vi "AlliGator Highlight Phasor ROI in Original Image v3.vi"(0 "AlliGator IV DVR in":refnum<data-value>, 1 "Image Color Scale Information":T2, 2 "Temp Overlay?":bool, 5 "Source Image Display":T1, 7 "Phasor Plot Image":T1, 9 "Phasor Plot ROI":T3, 11 "Error In":errorcluster, 12 "Overlay Color":u32(colorbox)) -> (4 "AlliGator IV DVR out":refnum<data-value>, 6 "Source Image Display out":T1, 8 "Phasor Plot Image Out":T1, 14 "CPU (s)":dbl, 15 "Error Out":errorcluster)   [LabVIEW 2021, in "AlliGator Source Image.lvlib"]
doc: "Compute and overlays the selected Phasor Plot ROI's pixels in the Source Image."
uses:
  AlliGator Source Image.lvlib
  AlliGator Internal Variables v2.ctl
  <vilib>/vision/Image Controls.llb/IMAQ Image.ctl
  AlliGator Gate Image Set.ctl
  AlliGator FLI Dataset Type.ctl
  AlliGator Data Series Type.ctl
  AlliGator Dataset Channel.ctl
  AlliGator Gate Arithmetic.ctl
  AlliGator Displayed Image.ctl
  Image/Named ROI Description.ctl
  AlliGator Decay Metadata v3.ctl
  AlliGator Decay Background Subtraction Info.ctl
  AlliGator Baseline Subtraction Method.ctl
  Graphs/XY Graph/XY Graph Plot Shift Parameters.ctl
  Graphs/XY Graph/XY Graph Plot Shift Method.ctl
  AlliGator Decay Extrapolation Parameters.ctl
  Phasor/Calibration Phasor (m, phi).ctl
  Phasor/Phasor Reference Series.ctl
  Phasor/Phasor Calibration Map v2.ctl
  Phasor/Phasor (g, s).ctl
  AlliGator Raw Phasor Plot Data v4.ctl
  Phasor/Phasor Standard Deviation Options.ctl
  AlliGator Phasor Multi-Harmonic Data.ctl
  Phasor/Phasor Harmonic Data.ctl
  AlliGator Decay Fit Options & Parameters v2.ctl
  Fits/IRF(X)PSED/Decay Fit Options v2.ctl
  Fits/Decay Convolution/Decay Model.ctl
  Fits/Residual Type.ctl
  Fits/IRF(X)PSED/Fit Weights Type.ctl
  Fits/Non-linear Fitting Method v2.ctl
  Fits/Fit Calculation Method.ctl
  Fits/Non-linear Fitting Algorithm.ctl
  AlliGator Decay Fit Parameter Constraints 2.ctl
  Fits/IRF(X)PSED/Decay Fit Parameters In List.ctl
  Fits/IRF(X)PSED/MLE Baseline Offset Type.ctl
  AlliGator Decay Preprocessing Parameters.ctl
  Fits/IRF(X)PSED/Decay Fit Parameters & Derived Quantities List.ctl
  Image/Image Color Scale Information.ctl
  AlliGator Variables List.ctl
  AlliGator Phasor Plot Reference Points.ctl
  AlliGator ROI Manager Actions.ctl
  Palette/Image Palette Information.ctl
  Image/Image Display Palette Type.ctl
  AlliGator Settings List.ctl
  9cfa6bdc-d1e0-4e6c-94b8-050a3d16fc11.vi
  Variant/Variant to Data/Variant to Boolean.vi
  Image/Image Get Pixel Color.vi
  Image/Adjust Pixel Overlay Brightness.vi
  <vilib>/vision/NI_Vision_Development_Module.lvlib
  AlliGator Globals, Variables & Constants.lvlib
  AlliGator Phasor Ratio.lvlib
  Error/Error.lvlib
  AlliGator Settings.lvlib
  Variant/Variant to Data/Variant to Data.lvlib
  Time/Time.lvlib
  AlliGator ROIs.lvlib
  Utilities/Utilities.lvlib
  Image/Image.lvlib
  Palette/Palette.lvlib
  Variant/Variant to Data/Variant to U16.vi
  Phasor/Phasor.lvlib
  AlliGator Decay Preprocessing.lvlib
  Graphs/XY Graph/XY Graph Add-Ons.lvlib
  AlliGator Phasor Graph.lvlib
  AlliGator Files.lvlib
  AlliGator Phasor Plot.lvlib
  AlliGator Internal Variables.lvlib
  Fits/Fits.lvlib
  AlliGator Decay Fit.lvlib
  AlliGator Decay Fit Parameter Map.lvlib
  AlliGator Dual-Channel Datasets.lvlib
panel:
  in  "Image Color Scale":dbl(ramp)
  # "see the AlliGator License on the block diagram (Ctrl+E or Window:Show Block Diagram)"
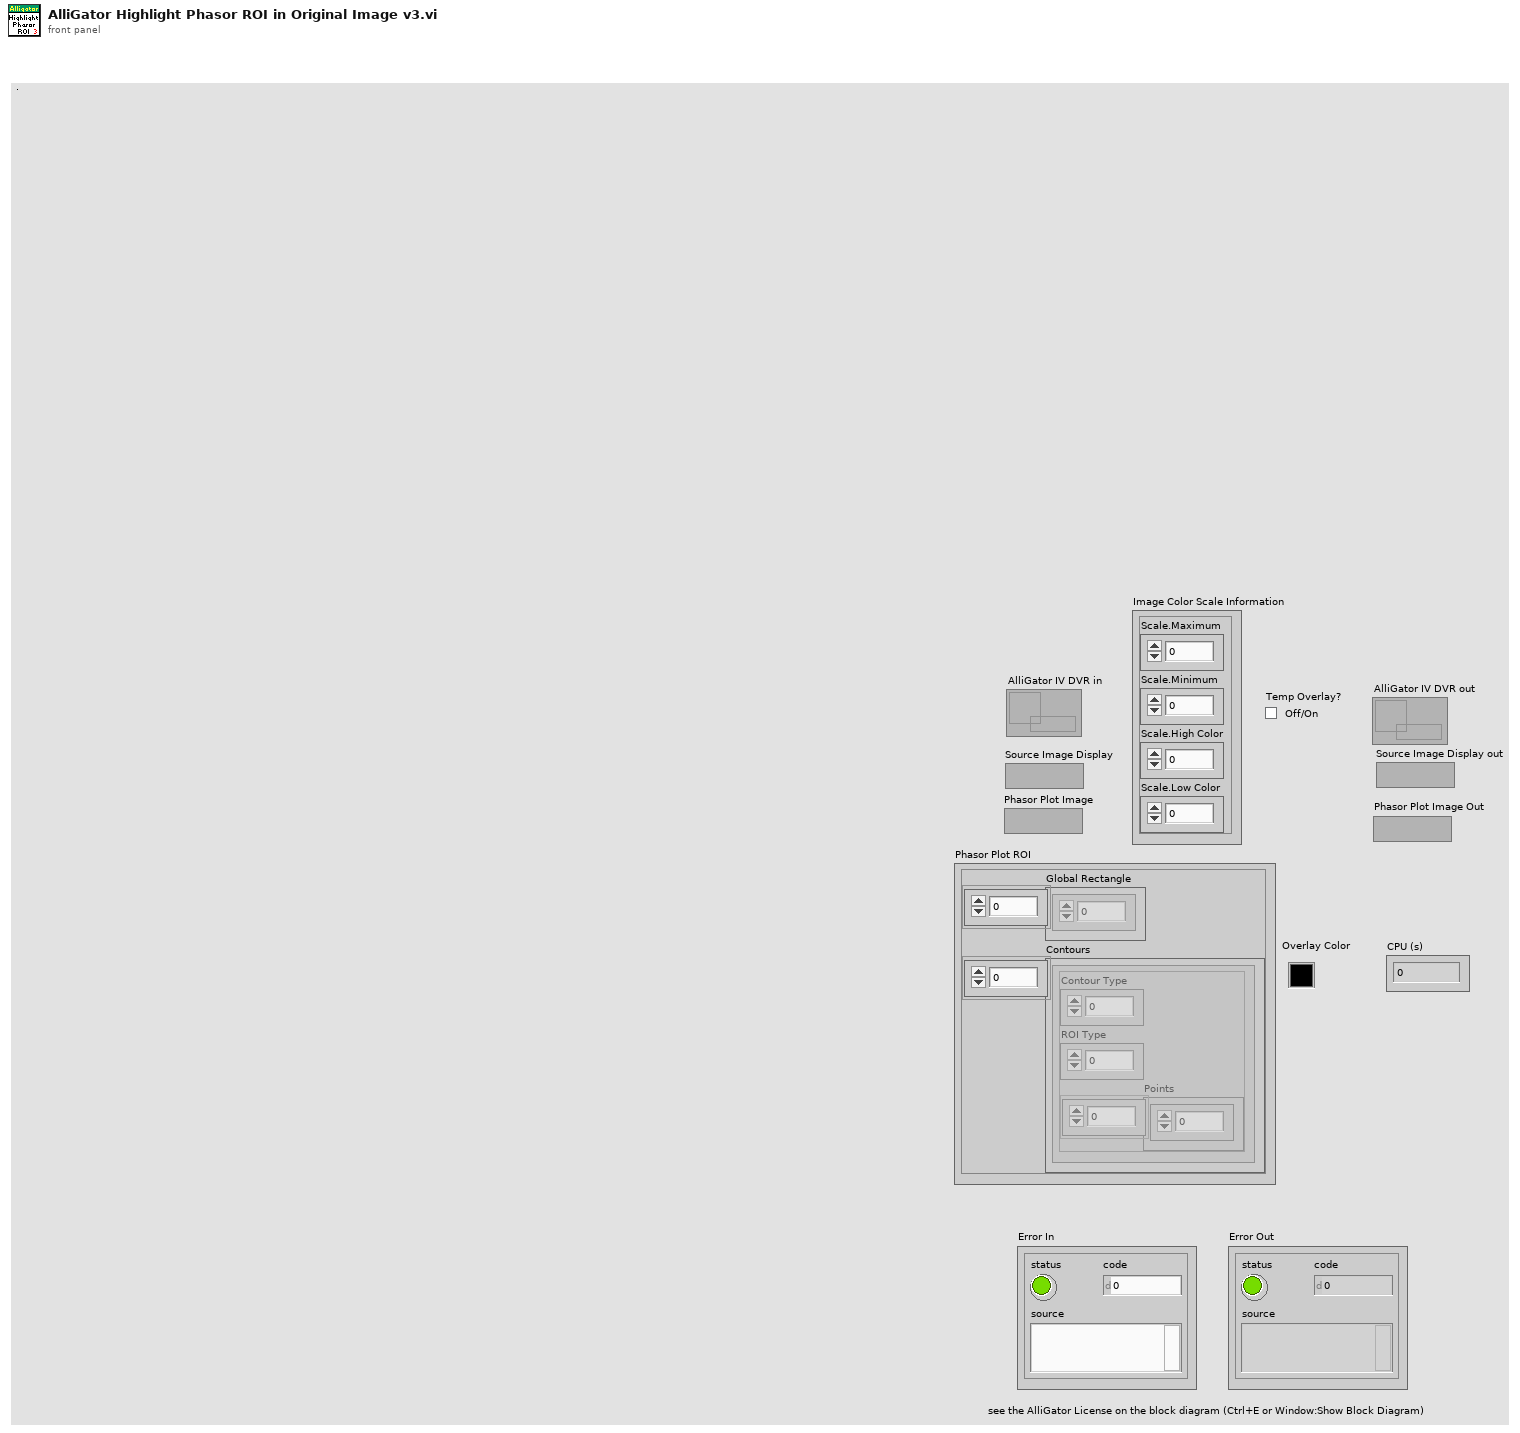
[diagram p1: front panel]
types:
  T1 = typedef "IMAQ Image.ctl" = refnum<image>
  T2 = typedef "Image.lvlib/Image Color Scale Information.ctl" = cluster{"Scale.Maximum":dbl, "Scale.Minimum":dbl, "Scale.High Color":u32, "Scale.Low Color":u32}
  T3 = cluster{"Global Rectangle":i32[], "Contours":cluster{"Contour Type":u32, "ROI Type":u32, "Points":i32[]}[]}
  T4 = typedef "AlliGator Settings.lvlib/AlliGator Settings List.ctl" = enum16{"GUI:Visible Settings Tab", "GUI:Last Run Version", "Source Image:Use Image Histogram for Contrast", "Source Image:Low Count Pixels Rejection Options", "Source Image:High Count Pixels Rejection Options", "Source Image:Use Image Brightness", "Source Image:Blend Overlay with Image Background", "Source Image:Use Fixed ROI Diameter", "Source Image:ROI Diameter", "Source Image:ROI Center Color", "Source Image:Peak Threshold", "Source Image:Intensity Threshold", "Source Image:Image Binning Options", "Source Image:Image Smoothing Options", "Source Image:Image Histogram Active", "Source Image:Invert Binary Mask", "Source Image:Hot Pixel Removal", "Source Image:Overlay Analyzed ROI Center", "Source Image:Auto-Adjust Contrast", "Source Image:Histogram Lower Percentile", "Source Image:Histogram Upper Percentile", "Source Image:Save Source Image", "Source Image:Scale Bar Options", "Source Image:Image Resolution (Pixel Size)", "Source Image:Flatfield Correction", "Source Image:Show Dead Left Columns Correction", "Source Image:Dead Left Columns Correction", "Source Image:Image Pre-Processing Operations Order", "Data Information:Gate Width", "Data Information:Nanotime Gate Separation", "Data Information:Macrotime Gate Separation", "Data Information:Gate Step", "Data Information:# Gates", "Data Information:Gate Image Exposure", "Data Information:Gate Image Integration", "Data Information:Gates to Skip", "Data Information:Gates to Keep", "Data Information:Define Gates to", "Data Information:Channel Name", "Data Information:Available Channel Names", "Data Information:Channel Arithmetic", "Data Information:Background File Subtraction", "Data Information:Background File", "Data Information:Background Scaling Factor", "Data Information:Background Pile-up Correction", "Data Information:Background Pixel Well Capacity", "Data Information:Laser Period", "Data Information:SYNC Period", "Data Information:Pile-up Correction", "Data Information:Pixel Well Capacity", "Data Information:Dataset Scaling Factor", "Fluorescence Decay_Decay Pre-Processing:Reverse Gates", "Fluorescence Decay_Decay Pre-Processing:Verbose Decay Pre-Processing", "Fluorescence Decay_Decay Pre-Processing:Use Decay Pre-Processing", "Fluorescence Decay_Decay Pre-Processing:Background Subtraction", "Fluorescence Decay_Decay Pre-Processing:Background Definition Range", "Fluorescence Decay_Decay Pre-Processing:Baseline Subtraction Method", "Fluorescence Decay_Decay Pre-Processing:Decay Pre-Processing Operations Order", "Fluorescence Decay_Decay Pre-Processing:Smoothing Parameter", "Fluorescence Decay_Decay Pre-Processing:Shift Decay", "Fluorescence Decay_Decay Pre-Processing:Decay Shift Parameters", "Fluorescence Decay_Decay Pre-Processing:Fold Decay", "Fluorescence Decay_Decay Pre-Processing:# Folds", "Fluorescence Decay_Decay Pre-Processing:1-Normalize Decay", "Fluorescence Decay_Decay Pre-Processing:[0-1]-Normalize Decay", "Fluorescence Decay_Decay Pre-Processing:Smoothen Decay", "Fluorescence Decay_Decay Pre-Processing:Extrapolate Decay", "Fluorescence Decay_Decay Pre-Processing:Use Periodicity", "Fluorescence Decay_Decay Pre-Processing:Use Cursors", "Fluorescence Decay_Decay Pre-Processing:Tail Fraction", "Fluorescence Decay_Decay Pre-Processing:Head Fraction", "Fluorescence Decay_Decay Pre-Processing:Additional Points", "Fluorescence Decay_Decay Pre-Processing:Straighten Decay", "Fluorescence Decay_Decay Pre-Processing:Constant Background", "Fluorescence Decay_Decay Pre-Processing:Pixel-Normalize Decay", "Fluorescence Decay_Advanced Analysis:Extract IRF instead of Decay", "Fluorescence Decay_Advanced Analysis:IRF Extraction Options", "Fluorescence Decay_Advanced Analysis:IRF Optimization Options", "Fluorescence Decay_Advanced Analysis:Square Pulse Options", "Fluorescence Decay_Advanced Analysis:IRF Order", "Fluorescence Decay_Advanced Analysis:IRF Time Constants", "Fluorescence Decay_Advanced Analysis:Wavelet Analysis Options", "Fluorescence Decay_Advanced Analysis:Average Lifetime Options", "Fluorescence Decay_Fit Options:Fit Options", "Fluorescence Decay_Fit Options:Use Legacy Fitting Approach", "Fluorescence Decay_Fit Options:Use Data Information Laser Period", "Fluorescence Decay_Fit Parameters:Displayed Fit Parameters", "Fluorescence Decay_Fit Parameters:Fit Parameter Constraints", "Fluorescence Decay_Fit Parameters:Export Tabulated Results", "Fluorescence Decay_Fit Parameters:MLE Baseline Offset Type", "Fluorescence Decay_Fit Parameters:MLE Baseline Offset", "Fluorescence Decay_Fit Parameters:Guess Parameter Names", "Fluorescence Decay_Fit Parameters:Guess Parameter Values", "Fluorescence Decay_Fit Parameters:Guess Parameters Options", "Fluorescence Decay_Styles:Show Last Decay Only", "Fluorescence Decay_Styles:Decay Graph Color Array", "Fluorescence Decay:Decay Graph Active", "Fluorescence Decay Statistics:Min Peak Value", "Fluorescence Decay Statistics:Reject Low Decay Peak Pixels", "Fluorescence Decay Statistics:Reject High Decay Peak Pixels", "Fluorescence Decay Statistics:Max Peak Value", "Time Traces:Use File Timestamp", "Time Traces:Time Step", "Time Traces:Use Intensity Correction File", "Time Traces:Intensity Correction File", "Phasor Plot:Phasor Plot Smoothing Options", "Phasor Plot:Phasor Plot Size", "Phasor Plot:Phasor Plot Graphics Options", "Phasor Plot:Cumulative Phasor Plot", "Phasor Plot:Use Phasor Brightness", "Phasor Plot:Blend Overlay with Phasor Background", "Phasor Plot:Save Phasor Plot", "Phasor Plot:Show References", "Phasor Plot:Phasor Ratio Decay Range", "Phasor Plot:Exponential Fading", "Phasor Plot:Phasor Ratio Reference Colors", "Phasor Plot:Reference Radius", "Phasor Plot:Show Color Map Vertices", "Phasor Plot:Phasor Plot Active", "Phasor Plot:Phasor Ratio Color Map Type", "Phasor Plot:Phasor Ratio Color Map", "Phasor Plot:Phasor Ratio Display Range", "Phasor Plot:Selected Image ROI(s)", "Phasor Plot:All Image ROIs", "Phasor Plot:Selected Phasor Plot ROI(s)", "Phasor Plot:All Phasor Plot ROIs", "Phasor Plot:Phasor Ratio Color-Coded Quantity", "Phasor Plot:Store Phasor Harmonics", "Phasor Plot:Draw Reference Segment", "Phasor Plot:User-Defined Quantity", "Phasor Graph:Phasor Frequency", "Phasor Graph:Phasor Ratio Type", "Phasor Graph:Pixel-level Phasor Computation", "Phasor Graph:Save Phasor Graph", "Phasor Graph:Phasor Graph Active", "Phasor Graph:Phasor SDV Options", "Phasor Calibration:Use Backup Calibration if needed", "Phasor Graph:Define Shortest Lifetime as", "Phasor Calibration:Backup Calibration Type", "Phasor Calibration:Calibration Type", "Phasor Calibration:Calibration Lifetime", "Phasor Calibration:Calibration Map Algorithm", "Single-Exponential Phasor Locus (SEPL):Gate Parameters", "Single-Exponential Phasor Locus (SEPL):User-defined Gate", "Single-Exponential Phasor Locus (SEPL):User-defined IRF", "Single-Exponential Phasor Locus (SEPL):Phasor Parameters", "Single-Exponential Phasor Locus (SEPL):Decay & IRF Parameters", "Single-Exponential Phasor Locus (SEPL):Display Parameters", "Lifetime Analysis:Decay Analysis Parameters", "Lifetime Analysis:Lifetime Map Active", "Plugins:Python Settings", "Miscellaneous:Verbose Mode", "Miscellaneous:Beep after Script", "Miscellaneous:Saved Image File Format", "Miscellaneous:Exported Gate Image Settings", "Miscellaneous:Include Loading in Timing", "Miscellaneous:Verbose Settings Mode", "Miscellaneous:Histogram Options", "Miscellaneous:Beep on Error", "Miscellaneous:# Logical Processors Used", "Miscellaneous:ROI Description Max Characters", "Miscellaneous:Verbose Error Mode", "Miscellaneous:Transparent Mask Color"}
  T5 = typedef "Palette.lvlib/Image Palette Information.ctl" = cluster{"Palette Name [# Colors,int?,inv?]":string, "Palette Type":T6, "Palette Colors":u32[], "Interpolate?":bool}
  T6 = typedef "Image.lvlib/Image Display Palette Type.ctl" = u32
  T7 = typedef "AlliGator Globals, Variables & Constants.lvlib/AlliGator Variables List.ctl" = enum16{"---- GUI ----", "Initialization Status", "State Indicators Refnum", "Original AlliGator Menu Items", "Current Action Loop State", "Script in progress", "Playback", "Loop Playback", "Search ROI Used", "Search ROI", "Decay Graph Max Legend Size", "Intensity Graph Max Legend Size", "Decay Statistics Graph Max Legend Size", "Phasor Graph Max Legend Size", "Phasor Ratio Graph Max Legend Size", "Lifetime Graph Max Legend Size", "---- Files ----", "Export Dataset Frames as Individual Files", "Show Batch Export Help Balloons", "Frames in Dataset", "ptu File Frame Start Indices", "Current Frame in Dataset", "Current Frame Timestamp", "------ Python Plugins ------", "Python Plugins Information", "Python Session", "Valid Python Session?", "---- Source Image ----", "Dataset Loaded", "Dataset Metadata", "Dataset Channel", "Dataset Data Description", "Background Dataset Metadata", "Background Dataset Channel", "Background Dataset Data Description", "Background File Subtraction", "Background File Path", "Background File Pile-up Correction", "Background File Pixel Well Capacity", "Background File Scaling Factor", "Source Image ROIs", "Current Source Image ROI", "Source Image ROI Event Refnum", "X_Source Image Display Range", "X_Source Image Palette Information", "Source Image Palette List", "Source Image Scale", "Current Dataset Load Settings", "Source Image:ROI Overlay Color", "---- Image Profile Window ----", "Image Profile:Overlay ROI in Source Image", "Image Profile Window Event Refnum", "Image Profile:IntensityType", "Image Profile:Intensity Average Type", "Image Profile:Intensity-weighted SDV", "Image Profile:Box Profile Type", "Image Profile Window Open", "Image Profile:Plotted Fit Parameter", "X_Type of Displayed Image", "X_Time Gate Slider", "Dataset Path", "Source Image Overlay to Erase", "Is Displayed Image Accumulated", "White Light Image Modified", "Mask Image Modified", "Macrotime Gate Separation", "------ Phasor Graph -------", "Phasor Graph:Show Line", "---- Phasor Plot ---", "Phasor Plot Parameters Changed", "FLI Dataset Modified since last Phasor Plot Calculation", "Phasor Harmonics Data", "Selected Phasor Harmonics", "Phasor Harmonic Manager Event Refnum", "Phasor Plot ROIs", "Current Phasor Plot ROI", "Phasor Plot ROI Event Refnum", "Phasor Plot Image Reference Points", "Phasor Plot Computed", "Phasor Plot Palette Information", "Phasor Plot Palette List", "Phasor Ratio Palette Information", "Phasor Ratio Palette List", "Phasor Image Scale", "Phasor Plot Image Overlay to Erase", "Phasor Plot Image Elements to Update", "Current Phasor Plot Calculation Parameters", "Current Phasor Calibration Options", "Reset Cumulated Phasor Plot", "Phasor Ratio Reference 1", "Phasor Ratio Lifetime Reference 1", "Phasor Ratio Reference 1 Frequency", "Phasor Ratio Reference 2", "Phasor Ratio Lifetime Reference 2", "Phasor Ratio Reference 2 Frequency", "---- Decay Analysis ----", "Number of Selected Decays to Fit", "LS Fit Results", "LAR Fit Results", "BS Fit Results", "Last Decay Max - Min", "Best Fit Parameters", "Best Fit Parameter Names", "Actual Size X", "Actual Size Y", "Binning X", "Binning Y", "Actual # Gates", "Dataset Number", "Gates to...", "Gates Skipped", "Gates to keep", "Gate Step", "Gate Separation", "Reversed Gates", "Pile-up Correction", "Pixel Well Capacity", "Background Subtracted", "Background Subtraction Method", "Background Definition Range", "Background File (deprecated)", "Number of Dataset Accumulated", "Array of Accumulated Dataset Paths", "Do Averaged Datasets", "Destination File Path", "Process Plot Target", "Use 1/D as Phasor Frequency", "---- Decay Fit Parameter Map -----", "Decay Fit Parameter Map Palette Information", "Decay Fit Parameter Map Palette List", "Local Decay Graph Window Event Refnum", "------- Local Decay Window ---------", "Use normalized IRF for convolution", "----- Miscellaneous ----", "Skippable Dialog Windows Status"}
  T8 = typedef "AlliGator ROIs.lvlib/AlliGator ROI Manager Actions.ctl" = enum16{"Undefined", "Delete Current ROI", "Delete All Unselected ROIs", "Delete Multiple ROIs", "Delete All ROIs", "Swap ROIs", "Insert ROI", "Update Current ROI Descriptor", "Rename Current ROI", "Store New ROI", "Store Multiple ROIs", "Select Next ROI", "Select Previous ROI", "Find Selected ROI", "Show All ROIs", "Update ROI Manager Window", "Merge All ROIs", "Unmerge ROI", "Set Selected ROI by ID"}
  T9 = typedef "AlliGator Phasor Ratio.lvlib/AlliGator Phasor Plot Reference Points.ctl" = cluster{"O_h":dbl, "O_v":dbl, "1_h":dbl, "1_v":dbl}
  T10 = typedef "AlliGator Internal Variables.lvlib/AlliGator Internal Variables v2.ctl" = cluster{"Displayed Image":T1, "White Light Image":T1, "Mask Image":T1, "ROI Mask Image":T1, "Current Dataset Images 1":T11, "Background Dataset Images 1":T11, "Current Dataset Images 2":T11, "Background Dataset Images 2":T11, "Current Dataset Arithmetic Images":T11, "Accumulated Dataset Images 1":T11, "Accumulated Dataset Images 2":T11, "Accumulated Dataset Arithmetic Images":T11, "Phasor Plot Image":T1, "Decay Fit Parameter Map Image":T1, "Single Data Point Path":path, "White Light Image Path":path, "Mask Image Path":path, "Time-Series Folder":path, "[Time-Series Paths]":path[], "Current Dataset":i32, "Single Dataset Type":T12, "Current Folder":string, "AlliGator Data Series Type":T13, "# Datasets":i32, "Dual-Channel Dataset":bool, "Selected Channel Name":string, "Dataset Channel":T14, "Channel Arithmetic":T15, "Dual-Channel Background Dataset":bool, "Background Channel":T14, "Dual-Channel Accumulated Dataset":bool, "Start Time":dbl, "[Time-Series Timestamps]":dbl[], "[Intensity Corrections]":dbl[], "Time Series Script":bool, "Type of Displayed Image":T16, "Gate Image Slide":u16, "# Gates":i32, "ROIs":T17[], "ROI Decay":cluster{"t Array":dbl[], "I Array":dbl[]}, "Valid Decay":bool, "Decay  Metadata":T19, "Reference Decay Plot Name":string, "Reference Decay":cluster{"t Array":dbl[], "I Array":dbl[]}, "Decay Shift Plot":cluster{"Time Stamps":dbl[], "Decay Shifts":dbl[]}, "[Decays Max Values]":sgl[], "[Decays Min Values]":sgl[], "Calibration Phasor":T25, "Calibration Phasor Series":T26, "Phasor Calibration Map":T27, "Calibration Map MD5 Digest":string, "Last Raw Phasor":T28, "Last Calibrated Phasor":T28, "Last Calibrated Phasor SDV":T28, "Phasor Graph:Phasor Plot":cluster{"g Array":dbl[], "s Array":dbl[]}, "Phasor Graph:Phasor SDV Plot":cluster{"g Array":dbl[], "s Array":dbl[]}, "[Phasor Graph:Raw Phasor Plots]":T29[], "Phasor Plot locked to Ref 1":i32, "[Phasor Plot(s) locked to Ref 1]":i32[], "[Phasor Plot(s) locked to Ref 2]":i32[], "[Pixel Phasors]":T28[], "[[Sum Image]]":dbl[][], "[[CSG Phasors]]":csg[][], "[[Valid Pixel?]]":bool[][], "I/m/phi Dataset":cluster{"I/m/phi Dataset?":bool, "Base Frequency":dbl[unit], "Harmonic Orders":u8[]}, "Multi Phasor Plot Data":T31, "Decay Fit Options & Parameters":T33, "Fit Options: Decay Preprocessing Parameters":T44, "Fit Options: Reference Decay":cluster{"t Array":dbl[], "I Array":dbl[]}, "Is Full Image Parameters Map":bool, "Is Single-Pixels Parameters Map":bool, "NLSF Parameters Map X Resolution":i32, "NLSF Parameters Map Y Resolution":i32, "[Single Decay Fit Parameters]":dbl[], "Fit Model":T35, "[[Multiple Decays Fit Parameters]]":dbl[][], "[[Multiple Decays Fit Parameter SDVs]]":dbl[][], "[[IRFs]]":dbl[][], "IRF Array Time Axis":dbl[], "Decay Array Time Axis":dbl[], "[Decay Fit Parameter Names]":T45[], "[[Phasor Ratios]]":dbl[][], "[[Average Lifetimes]]":dbl[][], "Amplitude Weighted Average Lifetime":bool, "[Decay Sum]":dbl[], "[[User-defined Quantities]]":dbl[][], "User-defined Quantity":string}
  T11 = typedef "AlliGator Internal Variables.lvlib/AlliGator Gate Image Set.ctl" = cluster{"SGL Image Max":T1, "SGL Image Sum":T1, "SGL Gate Images":T1[], "SGL Image Min":T1}
  T12 = typedef "AlliGator Files.lvlib/AlliGator FLI Dataset Type.ctl" = enum16{"HDF5 FLI Dataset", "Gate Image Folder", ".sdt FLI Dataset (Becker & Hickl)", ".ptu FLI Dataset (PicoQuant)", "SS1 FLI Dataset", "SS2 FLI Dataset", "I/m/phi Dataset", ".bin FLI Dataset (PicoQuant Binned)", ".bin FLI Dataset (Piccolo Binned)"}
  T13 = typedef "AlliGator Files.lvlib/AlliGator Data Series Type.ctl" = enum16{"Not a Supported Series", "Gate Images Folder Series", "SwissSPAD 2 Dataset Series", "B&H FLI Dataset Series", "PicoQuant PTU FLI Dataset Series", "PicoQuant BIN FLI Dataset Series", "Piccolo hist BIN FLI Dataset Series", "HDF5 FLI Dataset Series"}
  T14 = typedef "AlliGator Dual-Channel Datasets.lvlib/AlliGator Dataset Channel.ctl" = enum16{"G2", "INT"}
  T15 = typedef "AlliGator Settings.lvlib/AlliGator Gate Arithmetic.ctl" = enum16{"None", "INT-G2", "G2/INT*<INT>", "(1 - G2/INT)*<INT>"}
  T16 = typedef "AlliGator Source Image.lvlib/AlliGator Displayed Image.ctl" = enum16{"Single Gate", "Sum of All Gates", "Max of All Gates", "Min of All Gates", "-", "White Ligth Image", "Mask Image"}
  T17 = typedef "Image.lvlib/Named ROI Description.ctl" = cluster{"ROI Descriptor":T18, "ROI Name":string, "Overlay Color":u32}
  T18 = typedef "ROI Descriptor" = cluster{"Global Rectangle":i32[], "Contours":cluster{"ID":enum32{"External", "Internal"}, "Type":u32, "Coordinates":i32[]}[]}
  T19 = typedef "AlliGator Phasor Graph.lvlib/AlliGator Decay Metadata v3.ctl" = cluster{"ROI Descriptor":T18, "ROI Center":cluster{"X":i32, "Y":i32}, "Decay Background Subtraction Info":T20, "Decay Reverted":bool, "Decay Smoothened":bool, "Decay Straightened":bool, "Fitted Tau (Decay Straightening)":dbl, "Decay Shift Parameters":T22, "Decay Shifted":bool, "Decay Extrapolated":bool, "Decay Extrapolation Parameters":T24, "Decay Normalized":bool, "Fold Decay":bool, "# Folds":u32}
  T20 = typedef "AlliGator Decay Analysis.lvlib/AlliGator Decay Preprocessing.lvlib/AlliGator Decay Background Subtraction Info.ctl" = cluster{"Laser Period":dbl[unit], "Gate Duration":dbl[unit], "Baseline Subtraction Method":T21, "Background Definition Range":cluster{"Min Gate":dbl[unit], "Max Gate":dbl[unit]}, "Total Intensity w/o Bkgd Subtraction":dbl, "Bkgd-subtracted Intensity (exp)":dbl, "# Data Points":i32, "Background/Gate":dbl, "Fitted Lifetime":dbl[unit], "Bkgd-subtracted Intensity (theo)":dbl}
  T21 = typedef "AlliGator Decay Analysis.lvlib/AlliGator Decay Preprocessing.lvlib/AlliGator Baseline Subtraction Method.ctl" = enum16{"Mean", "Min", "Square Gated Single-Exponential", "File", "Constant"}
  T22 = typedef "XY Graph Add-Ons.lvlib/XY Graph Plot Shift Parameters.ctl" = cluster{"Type":T23, "Shift":dbl[unit], "Threshold":dbl, "Rotate":bool}
  T23 = typedef "XY Graph Add-Ons.lvlib/XY Graph Plot Shift Method.ctl" = enum16{"Default", "CFD", "Threshold", "Cross-Correlation"}
  T24 = typedef "AlliGator Decay Analysis.lvlib/AlliGator Decay Preprocessing.lvlib/AlliGator Decay Extrapolation Parameters.ctl" = cluster{"Additional Points":u32, "Head Fraction":dbl, "Fitted Tau":dbl, "Use Periodicity":bool, "Use Cursors":bool, "Tail Fraction":dbl}
  T25 = typedef "Phasor.lvlib/Calibration Phasor (m, phi).ctl" = cluster{"m":dbl, "phi":dbl, "Phasor Frequency":dbl[unit], "Reference Lifetime":dbl[unit]}
  T26 = typedef "Phasor.lvlib/Phasor Reference Series.ctl" = cluster{"m Array":dbl[], "phi Array":dbl[], "Phasor Frequency":dbl[unit], "Calibration Lifetime":dbl[unit]}
  T27 = typedef "Phasor.lvlib/Phasor Calibration Map v2.ctl" = cluster{"Phasor Frequency":dbl[unit], "Calibration Lifetime":dbl[unit], "ROI Centers":cluster{"X":i32, "Y":i32}[], "ROI Descriptors":T18[], "Map Resolution X":i32, "Map Resolution Y":i32, "z Array":cdb[]}
  T28 = typedef "Phasor.lvlib/Phasor (g, s).ctl" = cluster{"g":dbl, "s":dbl}
  T29 = typedef "AlliGator Phasor Graph.lvlib/AlliGator Raw Phasor Plot Data v4.ctl" = cluster{"Phasor Plot Name":string, "Raw Phasor Plot":T28[], "Phasor Frequency":dbl[unit], "[Decay Metadata]":T19[], "Raw Phasor Plot SDV":T28[], "Phasor SDV Options":T30, "[Calibration Phasor]":T25[]}
  T30 = typedef "Phasor.lvlib/Phasor Standard Deviation Options.ctl" = cluster{"Compute Estimated SDV":bool, "# Replicas":u32, "Use Estimated Average Phasor":bool}
  T31 = typedef "AlliGator Phasor Plot.lvlib/AlliGator Phasor Multi-Harmonic Data.ctl" = cluster{"Base Frequency":dbl[unit], "# Harmonics":u8, "Harmonic Orders":u8[], "Phasor Plot Settings Checksum":u64, "Phasor Harmonic Data Array":T32[]}
  T32 = typedef "Phasor.lvlib/Phasor Harmonic Data.ctl" = cluster{"Phasor Harmonic Name":string, "Phasor Plot Settings Checksum":u64, "Phasor Frequency":dbl[unit], "Base Frequency":dbl[unit], "Harmonic Order":u8, "Phasor Plot Parameters":string, "Phasor Array [[CSG]]":csg[][], "Dataset File Path":path}
  T33 = typedef "AlliGator Decay Fit Parameter Map.lvlib/AlliGator Decay Fit Options & Parameters v2.ctl" = cluster{"SYNC Period":dbl[unit], "Fit Options":T34, "Fit Parameter Constraints":T41[], "MLE Baseline Offset":dbl, "MLE Baseline Offset Type":T43}
  T34 = typedef "Fits.lvlib/Decay Fit Options v2.ctl" = cluster{"Show Fit Residuals":bool, "Fit Model":T35, "Residual Type":T36, "Max Decay Percentile":dbl, "Min Decay Percentile":dbl, "Show Full Decay":bool, "Weights":T37, "Fitting Method":T38, "Compute Parameter Uncertainties":bool, "Periodic Boundaries":bool, "Model Calculation":T39, "Period":dbl[unit], "Termination Criteria":cluster{"Max Iterations":i32, "Max Function Calls":i32, "Max Time":dbl[unit], "Function Tolerance":dbl, "Parameter Tolerance":dbl, "Gradient Tolerance":dbl, "Min Lambda":dbl, "Max Lambda":dbl, "Initial Tick Count":u32}, "Offset Resolution":dbl[unit], "Use Local IRF":bool, "Fitting Algorithm":T40}
  T35 = typedef "Fits.lvlib/Decay Model.ctl" = enum16{"1-Exponential", "2-Exponentials"}
  T36 = typedef "Fits.lvlib/Residual Type.ctl" = enum16{"Standard", "Normalized", "Reduced"}
  T37 = typedef "Fits.lvlib/Fit Weights Type.ctl" = enum16{"Unweighted", "1/Variance", "Best of All"}
  T38 = typedef "Fits.lvlib/Non-linear Fitting Method v2.ctl" = enum16{"Least Square", "Least Absolute Residual", "Bisquare", "MLE", "-", "Best of All"}
  T39 = typedef "Fits.lvlib/Fit Calculation Method.ctl" = enum16{"Simulation", "Convolution", "Integration"}
  T40 = typedef "Fits.lvlib/Non-linear Fitting Algorithm.ctl" = enum16{"Levenberg-Marquardt", "Trust-Region Dogleg"}
  T41 = typedef "AlliGator Decay Analysis.lvlib/AlliGator Decay Fit.lvlib/AlliGator Decay Fit Parameter Constraints 2.ctl" = cluster{"Fit Parameter":T42, "Min Value":dbl, "Max Value":dbl, "Global":bool, "Used":bool}
  T42 = typedef "Fits.lvlib/Decay Fit Parameters In List.ctl" = enum16{"Offset", "Baseline", "A_1", "tau_1", "A_2", "tau_2"}
  T43 = typedef "Fits.lvlib/MLE Baseline Offset Type.ctl" = enum32{"Absolute", "Percentage"}
  T44 = typedef "AlliGator Decay Analysis.lvlib/AlliGator Decay Preprocessing.lvlib/AlliGator Decay Preprocessing Parameters.ctl" = cluster{"Background Subtraction":bool, "Straighten Decay":bool, "Reverse Gates":bool, "1-Normalized Decay":bool, "Smoothen Decay":bool, "Smoothing Parameter":dbl, "Shift Decay":bool, "Decay Shift Parameters":T22, "Extrapolate Decay":bool, "Additional Points":u32, "Head Fraction":dbl, "Pixel-Normalize Decay":bool, "Use Periodicity":bool, "Use Cursors":bool, "Tail Fraction":dbl, "Use Decay Pre-Processing":bool, "Fold Decay":bool, "# Folds":u32, "[0-1]-Normalized Decay":bool}
  T45 = typedef "Fits.lvlib/Decay Fit Parameters & Derived Quantities List.ctl" = enum16{"Offset", "Baseline", "A_1", "tau_1", "A_2", "tau_2", "<tau>_a", "f1_a", "f2_a", "<tau>_i", "f1_i", "f2_i", "-", "R^2", "Chi^2"}
  T46 = typedef "Image Type" = u32
  T47 = cluster{"Red (or Hue) value":u8, "Green (or Sat) value":u8, "Blue (or Light or Val) value":u8}
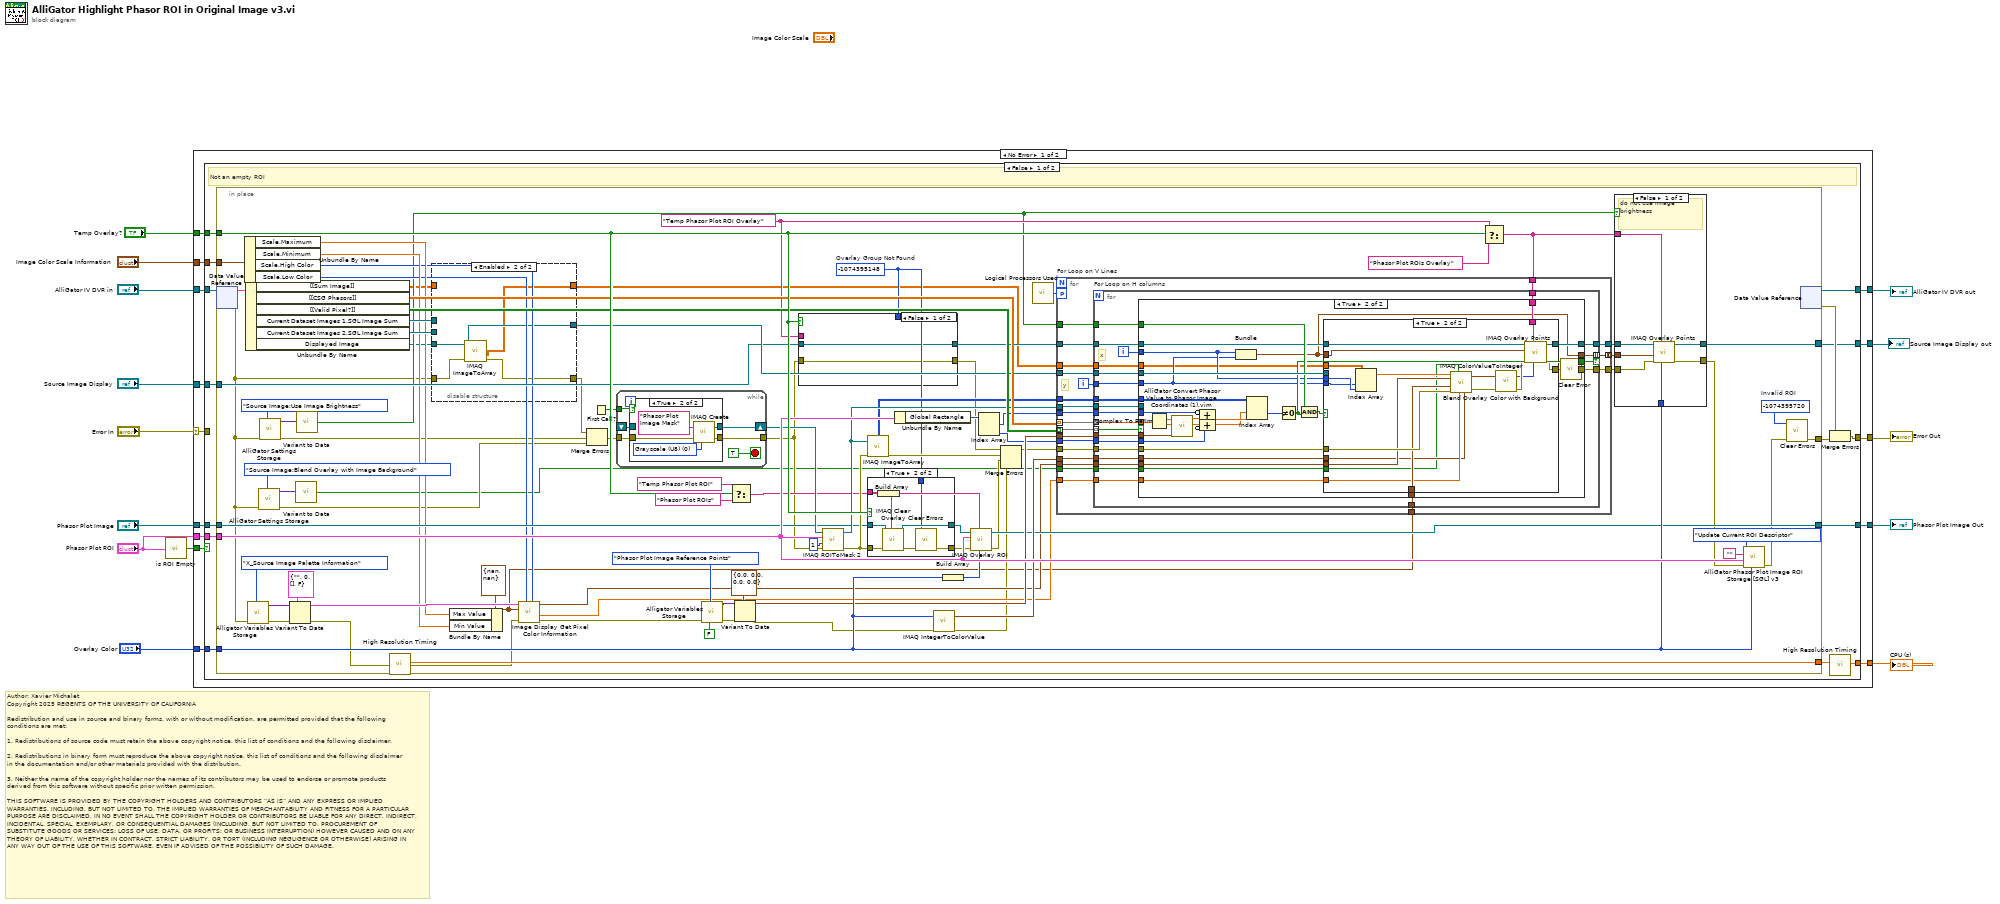
[diagram p0: block diagram]
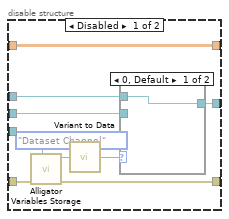
[diagram p5: hidden frame]
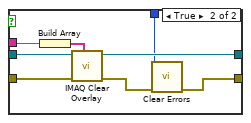
[diagram p8: hidden frame]
diagram:
  # "Author: Xavier Michalet\nCopyright 2025 REGENTS OF THE UNIVERSITY OF CALIFORNIA\n\nRedistribution and use in source and binary forms, with or without modification, are permitted provided that the following conditions are met:\n\n1. Redistributions of source code must retain the above copyright notice, this list of conditions and the following disclaimer.\n\n2. Redistributions in binary form must reproduce the above copyright notice, this list of conditions and the following disclaimer in the documentation and/or other materials provided with the distribution.\n\n3. Neither the name of the copyright holder nor the names of its contributors may be used to endorse or promote products derived from this software without specific prior written permission.\n\nTHIS SOFTWARE IS PROVIDED BY THE COPYRIGHT HOLDERS AND CONTRIBUTORS “AS IS” AND ANY EXPRESS OR IMPLIED WARRANTIES, INCLUDING, BUT NOT LIMITED TO, THE IMPLIED WARRANTIES OF MERCHANTABILITY AND FITNESS FOR A PARTICULAR PURPOSE ARE DISCLAIMED. IN NO EVENT SHALL THE COPYRIGHT HOLDER OR CONTRIBUTORS BE LIABLE FOR ANY DIRECT, INDIRECT, INCIDENTAL, SPECIAL, EXEMPLARY, OR CONSEQUENTIAL DAMAGES (INCLUDING, BUT NOT LIMITED TO, PROCUREMENT OF SUBSTITUTE GOODS OR SERVICES; LOSS OF USE, DATA, OR PROFITS; OR BUSINESS INTERRUPTION) HOWEVER CAUSED AND ON ANY THEORY OF LIABILITY, WHETHER IN CONTRACT, STRICT LIABILITY, OR TORT (INCLUDING NEGLIGENCE OR OTHERWISE) ARISING IN ANY WAY OUT OF THE USE OF THIS SOFTWARE, EVEN IF ADVISED OF THE POSSIBILITY OF SUCH DAMAGE."
  n1 = call "is ROI Empty.vi"("Current ROI Descriptor"="Phasor Plot ROI") -> ("Empty ROI?"=w9:bool)  [unwired: 8 in]
  n2 = case shown="No Error" "Error In" {
    selector: "Error In" -> [w15 w295]
    tunnel: "Overlay Color" -> [w28 _]
    tunnel: "AlliGator IV DVR in" -> [w27 w297]
    tunnel: [w26 w297] -> w12
    tunnel: [w25 w295] -> w11
    tunnel: "Temp Overlay?" -> [w24 _]
    tunnel: w9 -> [w23 _]
    tunnel: [w22 _] -> w8
    tunnel: "Phasor Plot ROI" -> [w21 _]
    tunnel: "Phasor Plot Image" -> [w20 w294]
    tunnel: [w19 w294] -> w5
    tunnel: "Source Image Display" -> [w18 w296]
    tunnel: [w17 w296] -> w3
    tunnel: "Image Color Scale Information" -> [w16 _]
    frame No Error {
      n3 = case shown="False" w23 {
        tunnel: w28 -> [w42 _]
        tunnel: w27 -> [w41 w293]
        tunnel: [w40 w293] -> w26
        tunnel: [w39 w290] -> w25
        tunnel: w24 -> [w37 _]
        tunnel: w20 -> [w36 w291]
        tunnel: w21 -> [w35 _]
        tunnel: [w33 _] -> w22
        tunnel: [w32 w291] -> w19
        tunnel: w18 -> [w31 w292]
        tunnel: [w30 w292] -> w17
        tunnel: w16 -> [w29 _]
        tunnel: w15 -> [_ w290]
        frame False {
          # "Not an empty ROI"
          n4 = in-place {
            in-place-border: w36 -> [w84]
            in-place-border: [w132] -> w43
            in-place-border: w42 -> [w121]
            in-place-border: [w131] -> w34
            in-place-border: w37 -> [w129]
            in-place-border: w35 -> [w128]
            in-place-border: [w83] -> w32
            in-place-border: w31 -> [w72]
            in-place-border: [w81] -> w30
            in-place-border: w29 -> [w63]
            w85 = -1074395148  # Overlay Group Not Found
            w93 = "Temp Phasor Plot ROI Overlay" ("Group")
            w125 = -1074395720  # Invalid ROI
            n5 = in-place-dvr #1(w41) -> (w130:T10, w52:errorcluster)
            n6 = Unbundle By Name(w63) -> ("Scale.Maximum"=w62:dbl, "Scale.Minimum"=w61:dbl, "Scale.High Color"=w60:u32, "Scale.Low Color"=w59:u32)
            n7 = Unbundle By Name(w130) -> ("[[Sum Image]]"=w47:dbl[][], "[[CSG Phasors]]"=w126:csg[][], "[[Valid Pixel?]]"=w127:bool[][], "Current Dataset Images 1.SGL Image Sum"=w123:T1, "Current Dataset Images 2.SGL Image Sum"=w122:T1, "Displayed Image"=w45:T1)
            n8 = call "Alligator Variables Storage.vi"("AlliGator Variable"=AlliGator_Variables_List."X_Source Image Palette Information" ("Alligator Variable"), "Error In"=w52) -> ("Error Out"=w78:errorcluster, "Data out"=w77:variant)  [unwired: 7 in, 1 out]
            n9 = call "AlliGator Settings Storage.vi"("AlliGator Settings List"=AlliGator_Settings_List."Source Image:Blend Overlay with Image Background", "Error In"=w52) -> ("Error Out"=w50:errorcluster, "Variant Data out"=w54:variant)  [unwired: 8 in]
            n10 = call "AlliGator Settings Storage.vi"("AlliGator Settings List"=AlliGator_Settings_List."Source Image:Use Image Brightness", "Error In"=w52) -> ("Error Out"=w56:errorcluster, "Variant Data out"=w58:variant)  [unwired: 8 in]
            n11 = Variant To Data(error in=w78, type=T5 {"Palette Name [# Colors,int?,inv?]"="", "Palette Type"=0, "Palette Colors"=[], "Interpolate?"=FALSE} ("Image Display Palette Information"), Variant=w77) -> (data=w75:T5, error out=w69:errorcluster)
            n12 = call-poly "Variant to Data.vi"("Variant"=w54) -> ("Value"=w48:bool)  [unwired: 8 in]
            n13 = call-poly "Variant to Data.vi"("Variant"=w58) -> ("Value"=w55:bool)  [unwired: 8 in]
            n14 = call "High Resolution Timing.vi"("Error In"=w69) -> ("elapsed (relative) seconds"=w131:dbl, "Error Out"=w68:errorcluster)  [unwired: 16 in, 1 out]
            n15 = disable-structure shown="Enabled" {
              disable-tunnel: [w250 w254] -> w124
              disable-tunnel: w123 -> [w249 _]
              disable-tunnel: w122 -> [w248 _]
              disable-tunnel: w52 -> [w244 w256]
              disable-tunnel: [w243 w255] -> w49
              disable-tunnel: w47 -> [w242 _]
              disable-tunnel: [w242 w253] -> w46
              disable-tunnel: w45 -> [_ w254]
              frame Disabled {
                n16 = call "Alligator Variables Storage.vi"("AlliGator Variable"=AlliGator_Variables_List."Dataset Channel" ("Alligator Variable"), "Error In"=w244) -> ("Error Out"=w243:errorcluster, "Data out"=w246:variant)  [unwired: 7 in, 1 out]
                n17 = call-poly "Variant to Data.vi"("Variant"=w246) -> ("U16 Value"=w245:u16)  [unwired: 8 in]
                n18 = case shown="0, Default" w245 {
                  tunnel: [w251 w252] -> w250
                  tunnel: w248 -> [_ w252]
                  tunnel: w249 -> [w251 _]
                  frame 0, Default {
                  }
                  frame 1 {
                  }
                }
              }
              frame Enabled {
                n19 = call "IMAQ ImageToArray"("error in (no error)"=w256, "Image"=w254) -> ("Image Pixels (Float)"=w253:sgl[][], "error out"=w255:errorcluster)  [unwired: 2 in, 3 out]
              }
            }
            n20 = Bundle By Name(cluster=cluster{"Min Value":sgl, "Max Value":sgl} {"Min Value"=nan, "Max Value"=nan} ("Image Display Range"), "Max Value"=w62, "Min Value"=w61) -> (w44:cluster{"Min Value":sgl, "Max Value":sgl})
            n21 = call "Image Display Get Pixel Color Information.vi"("Image High Color"=w60, "Image Low Color"=w59, "Error In"=w68, "Image Display Range"=w44, "Image Display Palette Information"=w75) -> ("Error Out"=w73:errorcluster, "Image Scale Factor (256 colors)"=w70:sgl, "1D Color Array"=w71:cluster{"Red":u8, "Green":u8, "Blue":u8}[])  [unwired: 3 in, 1 out]
            n22 = Merge Errors(w49, w56, w50) -> (w51:errorcluster)
            n23 = First Call?() -> (First Call?: T/F=w119:bool)
            n24 = while {
              tunnel: w119 -> [w282]
              tunnel: w51 -> [w281]
              shift-right: [w280] -> w89
              shift-left: _ -> [w278]
              tunnel: [w277] -> w80
              stop <- TRUE stop-if-true
              n25 = case shown="True" w282 {
                tunnel: w281 -> [w283 w288]
                tunnel: [w284 w287] -> w280
                tunnel: w278 -> [w284 _]
                tunnel: [w283 w286] -> w277
                frame False {
                }
                frame True {
                  w285 = T46 0 items=["Grayscale (U8)", "Grayscale (I16)", "Grayscale (SGL)", "Complex (CSG)", "RGB (U32)", "HSL (U32)", "RGB (U64)", "Grayscale (U16)"] ("Image Type")
                  n26 = call "IMAQ Create"("Image Name"="Phasor Plot Image Mask", "Image Type"=w285, "error in (no error)"=w288) -> ("New Image"=w287:T1, "error out"=w286:errorcluster)  [unwired: 2 in]
                }
              }
            }
            n27 = call "Alligator Variables Storage.vi"("Get(F)/Set"=FALSE, "AlliGator Variable"=AlliGator_Variables_List."Phasor Plot Image Reference Points" ("Alligator Variable"), "Error In"=w73) -> ("Error Out"=w114:errorcluster, "Data out"=w116:variant)  [unwired: 6 in, 1 out]
            n28 = Select(t="Temp Phasor Plot ROI" ("Group"), s=w129, f="Phasor Plot ROIs" ("Group")) -> (s? t:f=w86:string)
            n29 = Variant To Data(error in=w114, type=T9 {"O_h"=0.0, "O_v"=0.0, "1_h"=0.0, "1_v"=0.0} ("Phasor Plot Reference Points"), Variant=w116) -> (data=w113:T9, error out=w67:errorcluster)
            n30 = case shown="False" w129 {
              tunnel: w72 -> [w268 w276]
              tunnel: [w268 w275] -> w95
              tunnel: w80 -> [w267 w272]
              tunnel: [w267 w270] -> w94
              tunnel: w93 -> [_ w274]
              tunnel: w85 -> [_ w269]
              frame False {
              }
              frame True {
                n31 = Build Array(w274) -> (w273:string[])
                n32 = call "IMAQ Clear Overlay"("Groups"=w273, "error in (no error)"=w272, "Image"=w276) -> ("error out"=w271:errorcluster, "Image Out"=w275:T1)  [unwired: 7 in]
                n33 = call <vilib>:"Clear Errors.vi"("error in (no error)"=w271, "specific error code to clear (0: all)"=w269) -> ("error out"=w270:errorcluster)  [unwired: 4 in, 1 out]
              }
            }
            n34 = call "IMAQ ROIToMask 2"("error in (no error)"=w80, "Filling Value (255)"=1, "ROI Descriptor"=w128, "Image"=w89) -> ("error out"=w91:errorcluster, "Image Out"=w104:T1)  [unwired: 5 in, 1 out]
            n35 = call "IMAQ ImageToArray"("error in (no error)"=w91, "Image"=w104) -> ("error out"=w102:errorcluster, "Image Pixels (U8)"=w103:u8[][])  [unwired: 2 in, 3 out]
            n36 = case shown="True" w129 {
              tunnel: w84 -> [w258 w264]
              tunnel: [w258 w263] -> w92
              tunnel: w91 -> [w257 w262]
              tunnel: [w257 w260] -> w90
              tunnel: w86 -> [_ w265]
              tunnel: w85 -> [_ w259]
              frame False {
              }
              frame True {
                n37 = Build Array(w265) -> (w266:string[])
                n38 = call "IMAQ Clear Overlay"("Groups"=w266, "error in (no error)"=w262, "Image"=w264) -> ("error out"=w261:errorcluster, "Image Out"=w263:T1)  [unwired: 7 in]
                n39 = call <vilib>:"Clear Errors.vi"("error in (no error)"=w261, "specific error code to clear (0: all)"=w259) -> ("error out"=w260:errorcluster)  [unwired: 4 in, 1 out]
              }
            }
            n40 = Unbundle By Name(w128) -> ("Global Rectangle"=w101:i32[])
            n41 = call "IMAQ IntegerToColorValue"("error in (no error)"=w67, "U32 value"=w121) -> ("error out"=w66:errorcluster, "Color Value"=w111:T47)  [unwired: 3 in, 2 out]
            n42 = Build Array(w121) -> (w112:u32[])
            n43 = call "IMAQ Overlay ROI"("Colors (Green)"=w112, "Group"=w86, "error in (no error)"=w90, "ROI Descriptor"=w128, "Image"=w92) -> ("error out"=w82:errorcluster, "Image Out"=w83:T1)  [unwired: 5 in]
            n44 = Index Array(array=w101) -> (element #1=w100:i32, element #2=w99:i32)  [unwired: 2 in]
            n45 = Merge Errors(w94, w102, w82, w66) -> (w110:errorcluster)
            n46 = call "Logical Processors Used.vi"() -> ("# Logical Processor Used"=w98:i32)  [unwired: 6 in]
            n47 = Select(t=w93, s=w129, f="Phasor Plot ROIs Overlay" ("Group")) -> (s? t:f=w96:string)
            n48 = for "For Loop on V Lines" {
              tunnel: w126 -> [w163] mode=indexing
              tunnel: w104 -> [w161]
              tunnel: w113 -> [w160]
              tunnel: w100 -> [w159]
              tunnel: w99 -> [w158]
              tunnel: w124 -> [w157]
              tunnel: w111 -> [w156]
              tunnel: w96 -> [w155]
              tunnel: [w152] -> w109
              tunnel: [w151] -> w107 mode=concatenating
              tunnel: w110 -> [w154]
              tunnel: [w153] -> w108
              tunnel: w95 -> [w150]
              tunnel: w127 -> [w149] mode=indexing
              workers-P: w98 -> [_]
              tunnel: w55 -> [w148]
              tunnel: w103 -> [w147]
              tunnel: w46 -> [w146]
              tunnel: w71 -> [w145]
              tunnel: w70 -> [w144]
              tunnel: w48 -> [w143]
              tunnel: w44 -> [w142]
              i -> [w162]
              # "y"
              n49 = for "For Loop on H columns" {
                tunnel: w163 -> [w187] mode=indexing
                tunnel: w162 -> [w181]
                tunnel: w161 -> [w186]
                tunnel: w160 -> [w185]
                tunnel: w159 -> [w184]
                tunnel: w158 -> [w183]
                tunnel: w157 -> [w182]
                tunnel: w156 -> [w179]
                tunnel: w155 -> [w178]
                tunnel: [w177] -> w152
                tunnel: w148 -> [w176]
                tunnel: [w175] -> w151 mode=indexing if=w171
                tunnel: w154 -> [w172]
                tunnel: [w174] -> w153
                tunnel: w150 -> [w173]
                tunnel: w149 -> [w170] mode=indexing
                tunnel: w147 -> [w169]
                tunnel: w146 -> [w168]
                tunnel: w145 -> [w167]
                tunnel: w144 -> [w166]
                tunnel: w143 -> [w165]
                tunnel: w142 -> [w164]
                i -> [w180]
                # "x"
                n50 = case shown="True" w170 {
                  tunnel: w187 -> [_ w217]
                  tunnel: w186 -> [_ _]
                  tunnel: w185 -> [_ w215]
                  tunnel: w184 -> [_ w211]
                  tunnel: w183 -> [_ w210]
                  tunnel: w182 -> [_ w209]
                  tunnel: w181 -> [_ w197]
                  tunnel: w180 -> [_ w198]
                  tunnel: w179 -> [_ w208]
                  tunnel: w178 -> [_ w207]
                  tunnel: [w189 w205] -> w177
                  tunnel: w176 -> [_ w203]
                  tunnel: [_ w194] -> w175
                  tunnel: [w188 w202] -> w174
                  tunnel: w173 -> [w189 w201]
                  tunnel: w172 -> [w188 w200]
                  tunnel: [_ w199] -> w171
                  tunnel: w169 -> [_ w196]
                  tunnel: w168 -> [_ w195]
                  tunnel: w167 -> [_ w193]
                  tunnel: w166 -> [_ w192]
                  tunnel: w165 -> [_ w191]
                  tunnel: w164 -> [_ w190]
                  frame False {
                  }
                  frame True {
                    n51 = Complex To Re/Im(x + iy=w217) -> (x=w218:sgl, y=w216:sgl)
                    n52 = call "AlliGator Convert Phasor Value to Phasor Image Coordinates (1).vim"("Phasor Plot Reference Points"=w215, "Phasor s"=w216, "Phasor g"=w218) -> ("Phasor Plot y"=w220:dbl, "Phasor Plot x"=w213:dbl)  [unwired: 7 in]
                    n53 = Compound Arithmetic op=ADD(invert w211, w213) -> (w214:dbl)
                    n54 = Compound Arithmetic op=ADD(w220, invert w210) -> (w212:dbl)
                    n55 = Bundle(w198, w197) -> (w194:cluster{i32, i32})  [unwired: 1 in]
                    n56 = Index Array(array=w196, index (row)=w212, index (col)=w214) -> (element=w219:u8)
                    n57 = Not Equal To 0?(x=w219) -> (x != 0?=w199:bool)
                    n58 = Compound Arithmetic op=AND(w203, w199) -> (w204:bool)
                    n59 = case shown="True" w204 {
                      tunnel: w209 -> [_ _]
                      tunnel: w197 -> [_ w233]
                      tunnel: w198 -> [_ w234]
                      tunnel: w208 -> [_ w224]
                      tunnel: w194 -> [_ w239]
                      tunnel: w207 -> [_ w238]
                      tunnel: w200 -> [w222 w228]
                      tunnel: [w222 w237] -> w206
                      tunnel: [w221 w236] -> w205
                      tunnel: w201 -> [w221 w235]
                      tunnel: w195 -> [_ w232]
                      tunnel: w193 -> [_ w225]
                      tunnel: w192 -> [_ w226]
                      tunnel: w191 -> [_ w223]
                      tunnel: w190 -> [_ w227]
                      frame False {
                        # "do not use image brightness"
                      }
                      frame True {
                        n60 = Index Array(array=w232, index (row)=w233, index (col)=w234) -> (element=w229:sgl)
                        n61 = call "Blend Overlay Color with Background.vi"("Overlay Color Value"=w224, "Image Scale Factor"=w226, "Blend Overlay with Background"=w223, "error in (no error)"=w228, "Image Display Range"=w227, "Image Color Array"=w225, "Pixel Value"=w229) -> ("error out"=w231:errorcluster, "Scaled/Blended Overlay Color Value"=w230:T47)  [unwired: 3 in]
                        n62 = call "IMAQ ColorValueToInteger"("error in (no error)"=w231, "Color Value"=w230) -> ("error out"=w241:errorcluster, "U32 value"=w240:u32)  [unwired: 3 in, 2 out]
                        n63 = call "IMAQ Overlay Points"("Color"=w240, "Group"=w238, "error in (no error)"=w241, "Point"=w239, "Image"=w235) -> ("error out"=w237:errorcluster, "Image Out"=w236:T1)  [unwired: 5 in]
                      }
                    }
                    n64 = call "Clear Error.vi"("Error In"=w206) -> ("no Error Out"=w202:errorcluster)  [unwired: 8 in]
                  }
                }
              }
            }
            n65 = case shown="False" w55 {
              tunnel: w109 -> [w139 w141]
              tunnel: [w137 w141] -> w81
              tunnel: w96 -> [w138 _]
              tunnel: w108 -> [w136 w140]
              tunnel: [w135 w140] -> w65
              tunnel: w107 -> [w134 _]
              tunnel: w121 -> [w133 _]
              frame False {
                # "do not use image brightness"
                n66 = call "IMAQ Overlay Points"("Color"=w133, "Group"=w138, "error in (no error)"=w136, "Array of Points"=w134, "Image"=w139) -> ("error out"=w135:errorcluster, "Image Out"=w137:T1)  [unwired: 5 in]
              }
              frame True {
                # "already highlighted"
              }
            }
            n67 = call "AlliGator Phasor Plot Image ROI Storage [SGL] v3.vi"("Current Phasor Plot ROI Color"=w121, "Error In"=w65, "Current ROI Descriptor"=w128, "Default Name (\"ROI\")"="", "Action"=AlliGator_ROI_Manager_Actions."Update Current ROI Descriptor") -> ("Error Out"=w64:errorcluster)  [unwired: 1 in, 5 out]
            n68 = call <vilib>:"Clear Errors.vi"("error in (no error)"=w64, "specific error code to clear (0: all)"=w125) -> ("error out"=w132:errorcluster)  [unwired: 4 in, 1 out]
            n69 = in-place-dvr #1() -> (w40:refnum<data-value>, w38:errorcluster)  [unwired: 1 in]
          }
          n70 = Merge Errors(w38, w43) -> (w39:errorcluster)
          n71 = call "High Resolution Timing.vi"("relative seconds (NaN)"=w34) -> ("elapsed (relative) seconds"=w33:dbl)  [unwired: 16 in, 2 out]
        }
        frame True {
        }
      }
    }
    frame Error {
    }
  }
  "Error Out" <- w11
  "CPU (s)" <- w8
  "AlliGator IV DVR out" <- w12
  "Phasor Plot Image Out" <- w5
  "Source Image Display out" <- w3
